vi "General Control Settings Polymporhic.vi"(6 "Value":u8, 8 "error in (no error)":errorcluster, 10 "XML Elements":string) -> (0 "error out":errorcluster, 1 "Value Out":u8)   [LabVIEW 2014]
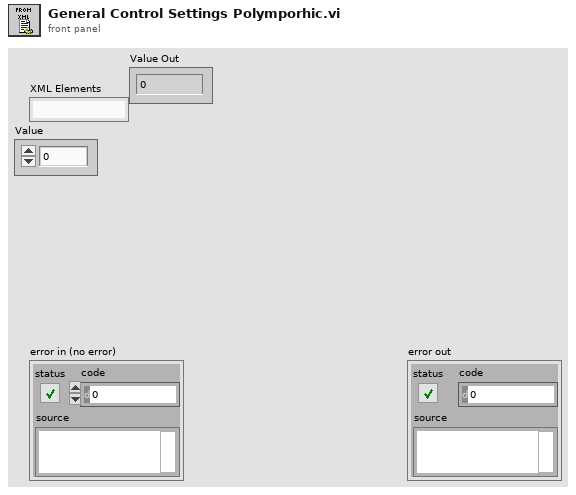
[diagram p1: front panel]
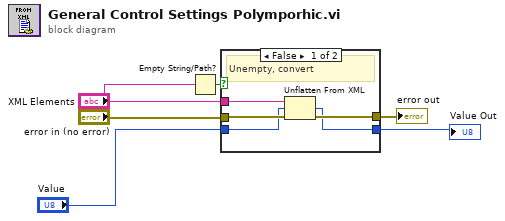
[diagram p0: block diagram]
diagram:
  n1 = Empty String/Path?(string/path="XML Elements") -> (empty?=w3:bool)
  n2 = case shown="False" w3 {
    tunnel: "error in (no error)" -> [w11 w12]
    tunnel: "Value" -> [w8 w13]
    tunnel: [w7 w13] -> w1
    tunnel: [w10 w12] -> w5
    tunnel: "XML Elements" -> [w9 _]
    frame False {
      # "Unempty, convert"
      n3 = Unflatten From XML(xml string=w9, type=w8, error in (no error)=w11) -> (value=w7:u8, error out=w10:errorcluster)
    }
    frame True {
      # "Empty, default values"
    }
  }
  "error out" <- w5
  "Value Out" <- w1
